vi "write_data_parameters.vi"(5 "Notes":string, 6 "data_type":T1, 7 "save_every_step?":bool, 8 "error in (no error)":errorcluster, 9 "xy_dims":u32[](array[numeric]), 10 "detector_data_dimensions":u32[](array[numeric]), 11 "scan_2d_hdf5_log in":refnum<class "scan_2d_hdf5_log.lvclass">) -> (0 "error out":errorcluster, 3 "scan_2d_hdf5_log out":refnum<class "scan_2d_hdf5_log.lvclass">)   [LabVIEW 2015, in "scan_2d_hdf5_log.lvclass"]
uses:
  scan_2d_hdf5_log.lvclass
  Detector_Class/detector/data_types_tdef.ctl
  scan_2d_hdf5_log.lvclass/scan_2d_hdf5_log.ctl
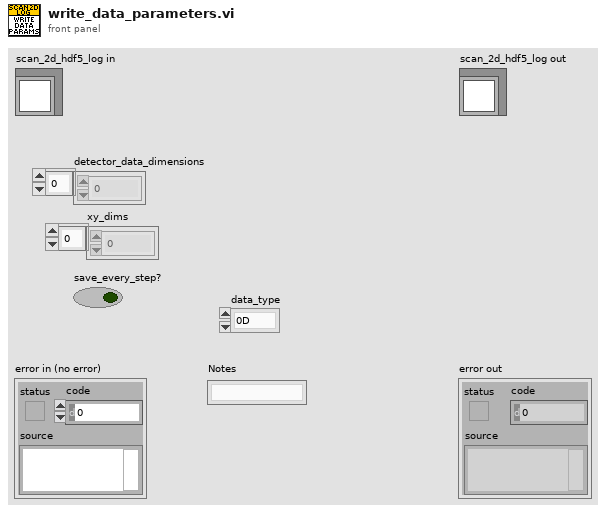
[diagram p1: front panel]
types:
  T1 = typedef "data_types_tdef.ctl" = enum16{"0D", "1D", "2D"}
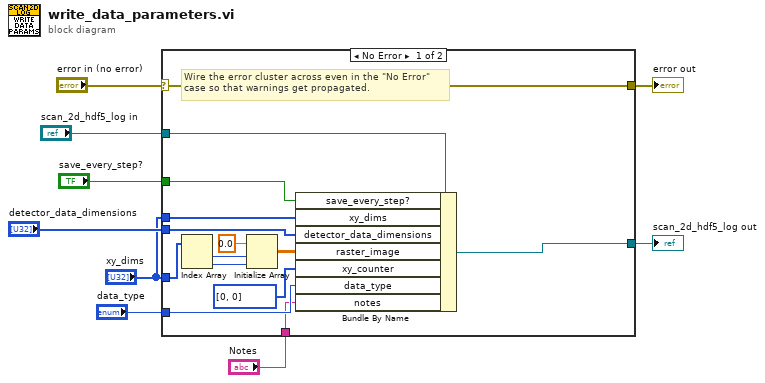
[diagram p0: block diagram]
diagram:
  n1 = case shown="No Error" "error in (no error)" {
    selector: "error in (no error)" -> [w23 w25]
    tunnel: [w23 w25] -> w8
    tunnel: [w18 w24] -> w6
    tunnel: "scan_2d_hdf5_log in" -> [w22 w24]
    tunnel: "save_every_step?" -> [w21 _]
    tunnel: "detector_data_dimensions" -> [w20 _]
    tunnel: "xy_dims" -> [w19 _]
    tunnel: "xy_dims" -> [w15 _]
    tunnel: "data_type" -> [w11 _]
    tunnel: "Notes" -> [w10 _]
    frame No Error {
      # "Wire the error cluster across even in the \"No Error\"\ncase so that warnings get propagated."
      n2 = Index Array(array=w15) -> (element #1=w17:u32, element #2=w14:u32)  [unwired: 2 in]
      n3 = Initialize Array(0.0 ("element"), w17, w14) -> (w13:dbl[][])
      n4 = Bundle By Name(cluster=w22, "save_every_step?"=w21, "xy_dims"=w19, "detector_data_dimensions"=w20, "raster_image"=w13, "xy_counter"=i32[] [0, 0], "data_type"=w11, "notes"=w10) -> (w18:refnum<class "scan_2d_hdf5_log.lvclass">)
    }
    frame Error {
    }
  }
  "error out" <- w8
  "scan_2d_hdf5_log out" <- w6
